vi "String_MeasParameters.vi"(11 "String":string="Measure 30 seconds or 10 points every 1 seconds, 10 averages") -> (1 "seconds":dbl=300.0, 2 "averages":i16=300, 3 "#points":i16=300, 5 "#seconds":dbl=300.0)   [LabVIEW 2017]
panel:
  # "Measure for 0.001 seconds or 0 points every 0.020 seconds, 10 averages"
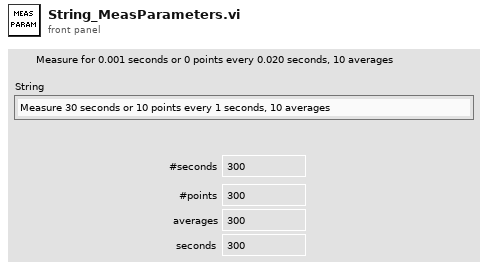
[diagram p1: front panel]
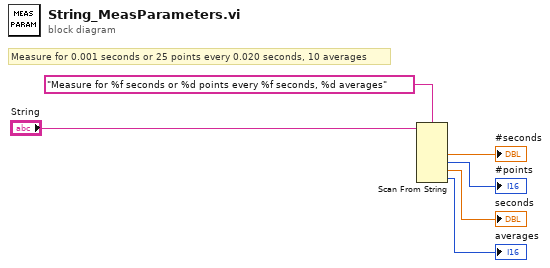
[diagram p0: block diagram]
diagram:
  # "Measure for 0.001 seconds or 25 points every 0.020 seconds, 10 averages"
  n1 = Scan From String(format string="Measure for %f seconds or %d points every %f seconds, %d averages", input string="String") -> (output 1=→"#seconds":dbl, output 2=→"#points":i16, output 3=→"seconds":dbl, output 4=→"averages":i16)  [unwired: 6 in, 3 out]
